vi "Initialize.vi"(8 "error in (no error)":errorcluster, 10 "Ctl Refnum":refnum<vi>, 11 "Boolean Object Position in":refnum<class "Boolean Object Position.lvclass">) -> (0 "error out":errorcluster, 3 "Boolean Object Position out":refnum<class "Boolean Object Position.lvclass">)   [LabVIEW 2018, in "Boolean Object Position.lvclass"]
uses:
  Boolean Object Position.lvclass
  Boolean Object Position.lvclass/Boolean Object Position.ctl
  Pane Object.lvclass/Pane Object Position.lvclass
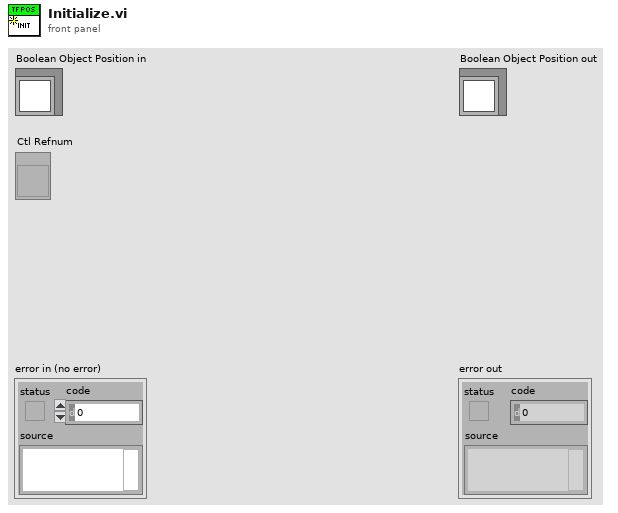
[diagram p1: front panel]
types:
  T1 = typedef "Pane Object Position.lvclass/Object Coordinates.ctl" = cluster{"Top":i32, "Right":i32, "Bottom":i32, "Left":i32}
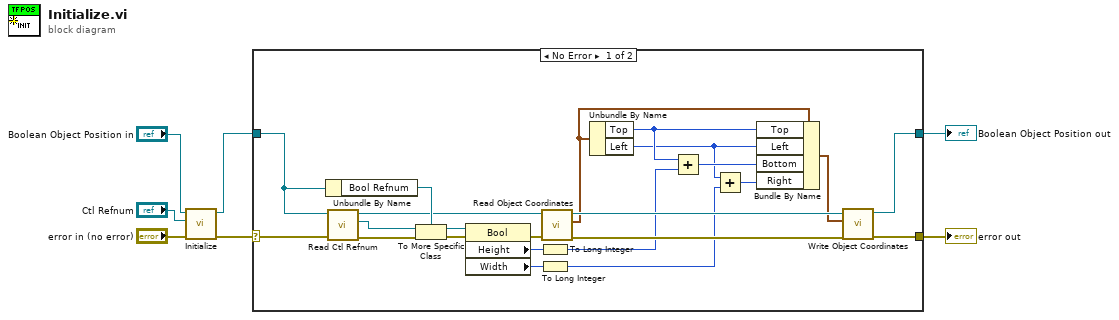
[diagram p0: block diagram]
diagram:
  n1 = call-parent "Initialize.vi"("error in (no error)"="error in (no error)", "Ctl Refnum"="Ctl Refnum", "Pane Object Position in"="Boolean Object Position in") -> ("error out"=w4:errorcluster, "Pane Object Position out"=w2:refnum<class "Boolean Object Position.lvclass">)  [unwired: 7 in]
  n2 = case shown="No Error" w4 {
    selector: w4 -> [w28 w32]
    tunnel: [w24 w32] -> w3
    tunnel: w2 -> [w23 w31]
    tunnel: [w25 w31] -> w1
    frame No Error {
      n3 = Unbundle By Name(w23) -> ("Bool Refnum"=w22:refnum<vi>)
      n4 = call-dynamic "Read Ctl Refnum.vi"("error in (no error)"=w28, "Pane Object Position in"=w23) -> ("error out"=w26:errorcluster, "Ctl Refnum"=w27:refnum<vi>, "Pane Object Position out"=w21:refnum<class "Boolean Object Position.lvclass">)  [unwired: 7 in]
      n5 = To More Specific Class(target class=w22, reference=w27, error in=w26) -> (specific class reference=w30:refnum<vi>, error out=w29:errorcluster)
      n6 = property class="Bool"(reference=w30, error in=w29) -> (error out=w19:errorcluster, "Height"=w17:u32, "Width"=w16:u32)  [unwired: 1 out]
      n7 = To Long Integer(number=w17) -> (32bit integer=w13:i32)
      n8 = To Long Integer(number=w16) -> (32bit integer=w9:i32)
      n9 = call-dynamic "Read Object Coordinates.vi"("error in (no error)"=w19, "Pane Object Position in"=w21) -> ("error out"=w18:errorcluster, "Object Coordinates"=w15:T1, "Pane Object Position out"=w20:refnum<class "Boolean Object Position.lvclass">)  [unwired: 7 in]
      n10 = Unbundle By Name(w15) -> ("Top"=w14:i32, "Left"=w10:i32)
      n11 = Add(x=w14, y=w13) -> (x+y=w12:i32)
      n12 = Add(x=w10, y=w9) -> (x+y=w11:i32)
      n13 = Bundle By Name(cluster=w15, "Top"=w14, "Left"=w10, "Bottom"=w12, "Right"=w11) -> (w8:T1)
      n14 = call-dynamic "Write Object Coordinates.vi"("error in (no error)"=w18, "Object Coordinates"=w8, "Pane Object Position in"=w20) -> ("error out"=w24:errorcluster, "Pane Object Position out"=w25:refnum<class "Boolean Object Position.lvclass">)  [unwired: 7 in]
    }
    frame Error {
    }
  }
  "error out" <- w3
  "Boolean Object Position out" <- w1
